vi "ATECC2 System Designer.vi"() -> ()   [LabVIEW 2023]
uses:
  <vilib>/ErrorRing/Error Ring.xnode
  Option Type Defs/Rack.ctl
  Option Type Defs/Full System Configuration.ctl
  Option Type Defs/Middle Rail.ctl
  Option Type Defs/Ballast.ctl
  Option Type Defs/Rear Panel IO Configuration.ctl
  Option Type Defs/Rear Panel IO.ctl
  Option Type Defs/Front Panel IO.ctl
  Option Type Defs/Front Door.ctl
  Option Type Defs/Miscellaneous Options.ctl
  <vilib>/Utility/sysdir.llb/System Directory Type.ctl
  Option Type Defs/Filler Panel Color.ctl
  Option Type Defs/Screw Types.ctl
  Option Type Defs/Accessories.ctl
  Option Type Defs/Parts List.ctl
panel:
  out "CSV-friendly String":string
  out "Parts List":T1[](array[typedef])
  out "Current Configuration":T2={"Rack"=enum."15U; 1-Phase; 16A; 100-240V", "Middle Rail"=enum."None", "Ballast"={"Main"=0, "Small"=0, "Side"=0}, "Front Panel I/O"={"EMO Button"=FALSE, "USB 3.0"=FALSE, "Display"=FALSE, "1st USB 2.0"=FALSE, "2nd USB 2.0"=FALSE, "Ethernet 3"=FALSE, "EMO Extension (3rd Party)"=FALSE, "EMO Extension (Rack In & Out)"=FALSE, "Aux Dual C13 QAC Outlets"=FALSE, "Residual-current Circuit Breaker"=FALSE, "Serial"=FALSE, "GPIB"=FALSE}, "Rear Panel I/O"={"Rear Panel I/O Configuration"=enum."Blank Panel", "EMO Button"=FALSE, "Power, Status & Banana Ground"=FALSE, "Ethernet 2"=FALSE, "Display"=FALSE, "USB 3.0"=FALSE, "DIO"=FALSE, "GPIB"=FALSE, "Aux Dual C13 QAC Outlets"=FALSE, "Residual-current Circuit Breaker"=FALSE, "Serial"=FALSE, "SMA"=FALSE}, "Miscellaneous Options"={"Eyebolts"=FALSE, "Tower Light"=FALSE, "Top/Side Monitor Mount Kit"=FALSE, "24\" Monitor"=FALSE, "Keyboard & Mouse"=FALSE, "Secondary Ethernet Switch"=FALSE, "Extra USB Hub"=FALSE, "USB-6509"=FALSE, "Front Door"=enum."38U (Solid) IG", "Primary Ethernet Switch"=enum."Item 0", "Use Posture"=enum."Item 0"}, "Accessories"={"Screw Type"=enum."10-32", "Cage Nuts & Screws"=0.0, "Filler Panel Color"=enum."Interface Gray", "1U"=0.0, "2U"=0.0, "3U"=0.0}} {"Ballast"."Side" max=5 step=1; "Ballast"."Small" max=5 step=1; "Ballast"."Main" max=5 step=1}
  in  "Full System Configuration":T2={"Rack"=enum."15U; 1-Phase; 16A; 100-240V", "Middle Rail"=enum."None", "Ballast"={"Main"=0, "Small"=0, "Side"=0}, "Front Panel I/O"={"EMO Button"=FALSE, "USB 3.0"=FALSE, "Display"=FALSE, "1st USB 2.0"=FALSE, "2nd USB 2.0"=FALSE, "Ethernet 3"=FALSE, "EMO Extension (3rd Party)"=FALSE, "EMO Extension (Rack In & Out)"=FALSE, "Aux Dual C13 QAC Outlets"=FALSE, "Residual-current Circuit Breaker"=FALSE, "Serial"=FALSE, "GPIB"=FALSE}, "Rear Panel I/O"={"Rear Panel I/O Configuration"=enum."Blank Panel", "EMO Button"=FALSE, "Power, Status & Banana Ground"=FALSE, "Ethernet 2"=FALSE, "Display"=FALSE, "USB 3.0"=FALSE, "DIO"=FALSE, "GPIB"=FALSE, "Aux Dual C13 QAC Outlets"=FALSE, "Residual-current Circuit Breaker"=FALSE, "Serial"=FALSE, "SMA"=FALSE}, "Miscellaneous Options"={"Eyebolts"=FALSE, "Tower Light"=FALSE, "Top/Side Monitor Mount Kit"=FALSE, "24\" Monitor"=FALSE, "Keyboard & Mouse"=FALSE, "Secondary Ethernet Switch"=FALSE, "Extra USB Hub"=FALSE, "USB-6509"=FALSE, "Front Door"=enum."38U (Solid) IG", "Primary Ethernet Switch"=enum."Item 0", "Use Posture"=enum."Item 0"}, "Accessories"={"Screw Type"=enum."10-32", "Cage Nuts & Screws"=0.0, "Filler Panel Color"=enum."Interface Gray", "1U"=0.0, "2U"=0.0, "3U"=0.0}} {"Ballast"."Side" max=5 step=1; "Ballast"."Small" max=5 step=1; "Ballast"."Main" max=5 step=1}
  # "1 DC 600 per AC PDU in system\n1 DC1200 per AC PDU in system"
  # "Rear panel I/O: Select one of the three major part numbers (fully, partial, blank).\nIf yoiu want custom, select the far right main panel and chose your piece-meal parts from the table below the Rear I/O secion."
  # "Front panel I/O just needs individual part numbers for I/O sub panels."
  # "The 15U version \"fully poipulate panel\" uses the DIO version, not the C13 version. If they wanbt the C13 version, they need to build it from a custom panel."
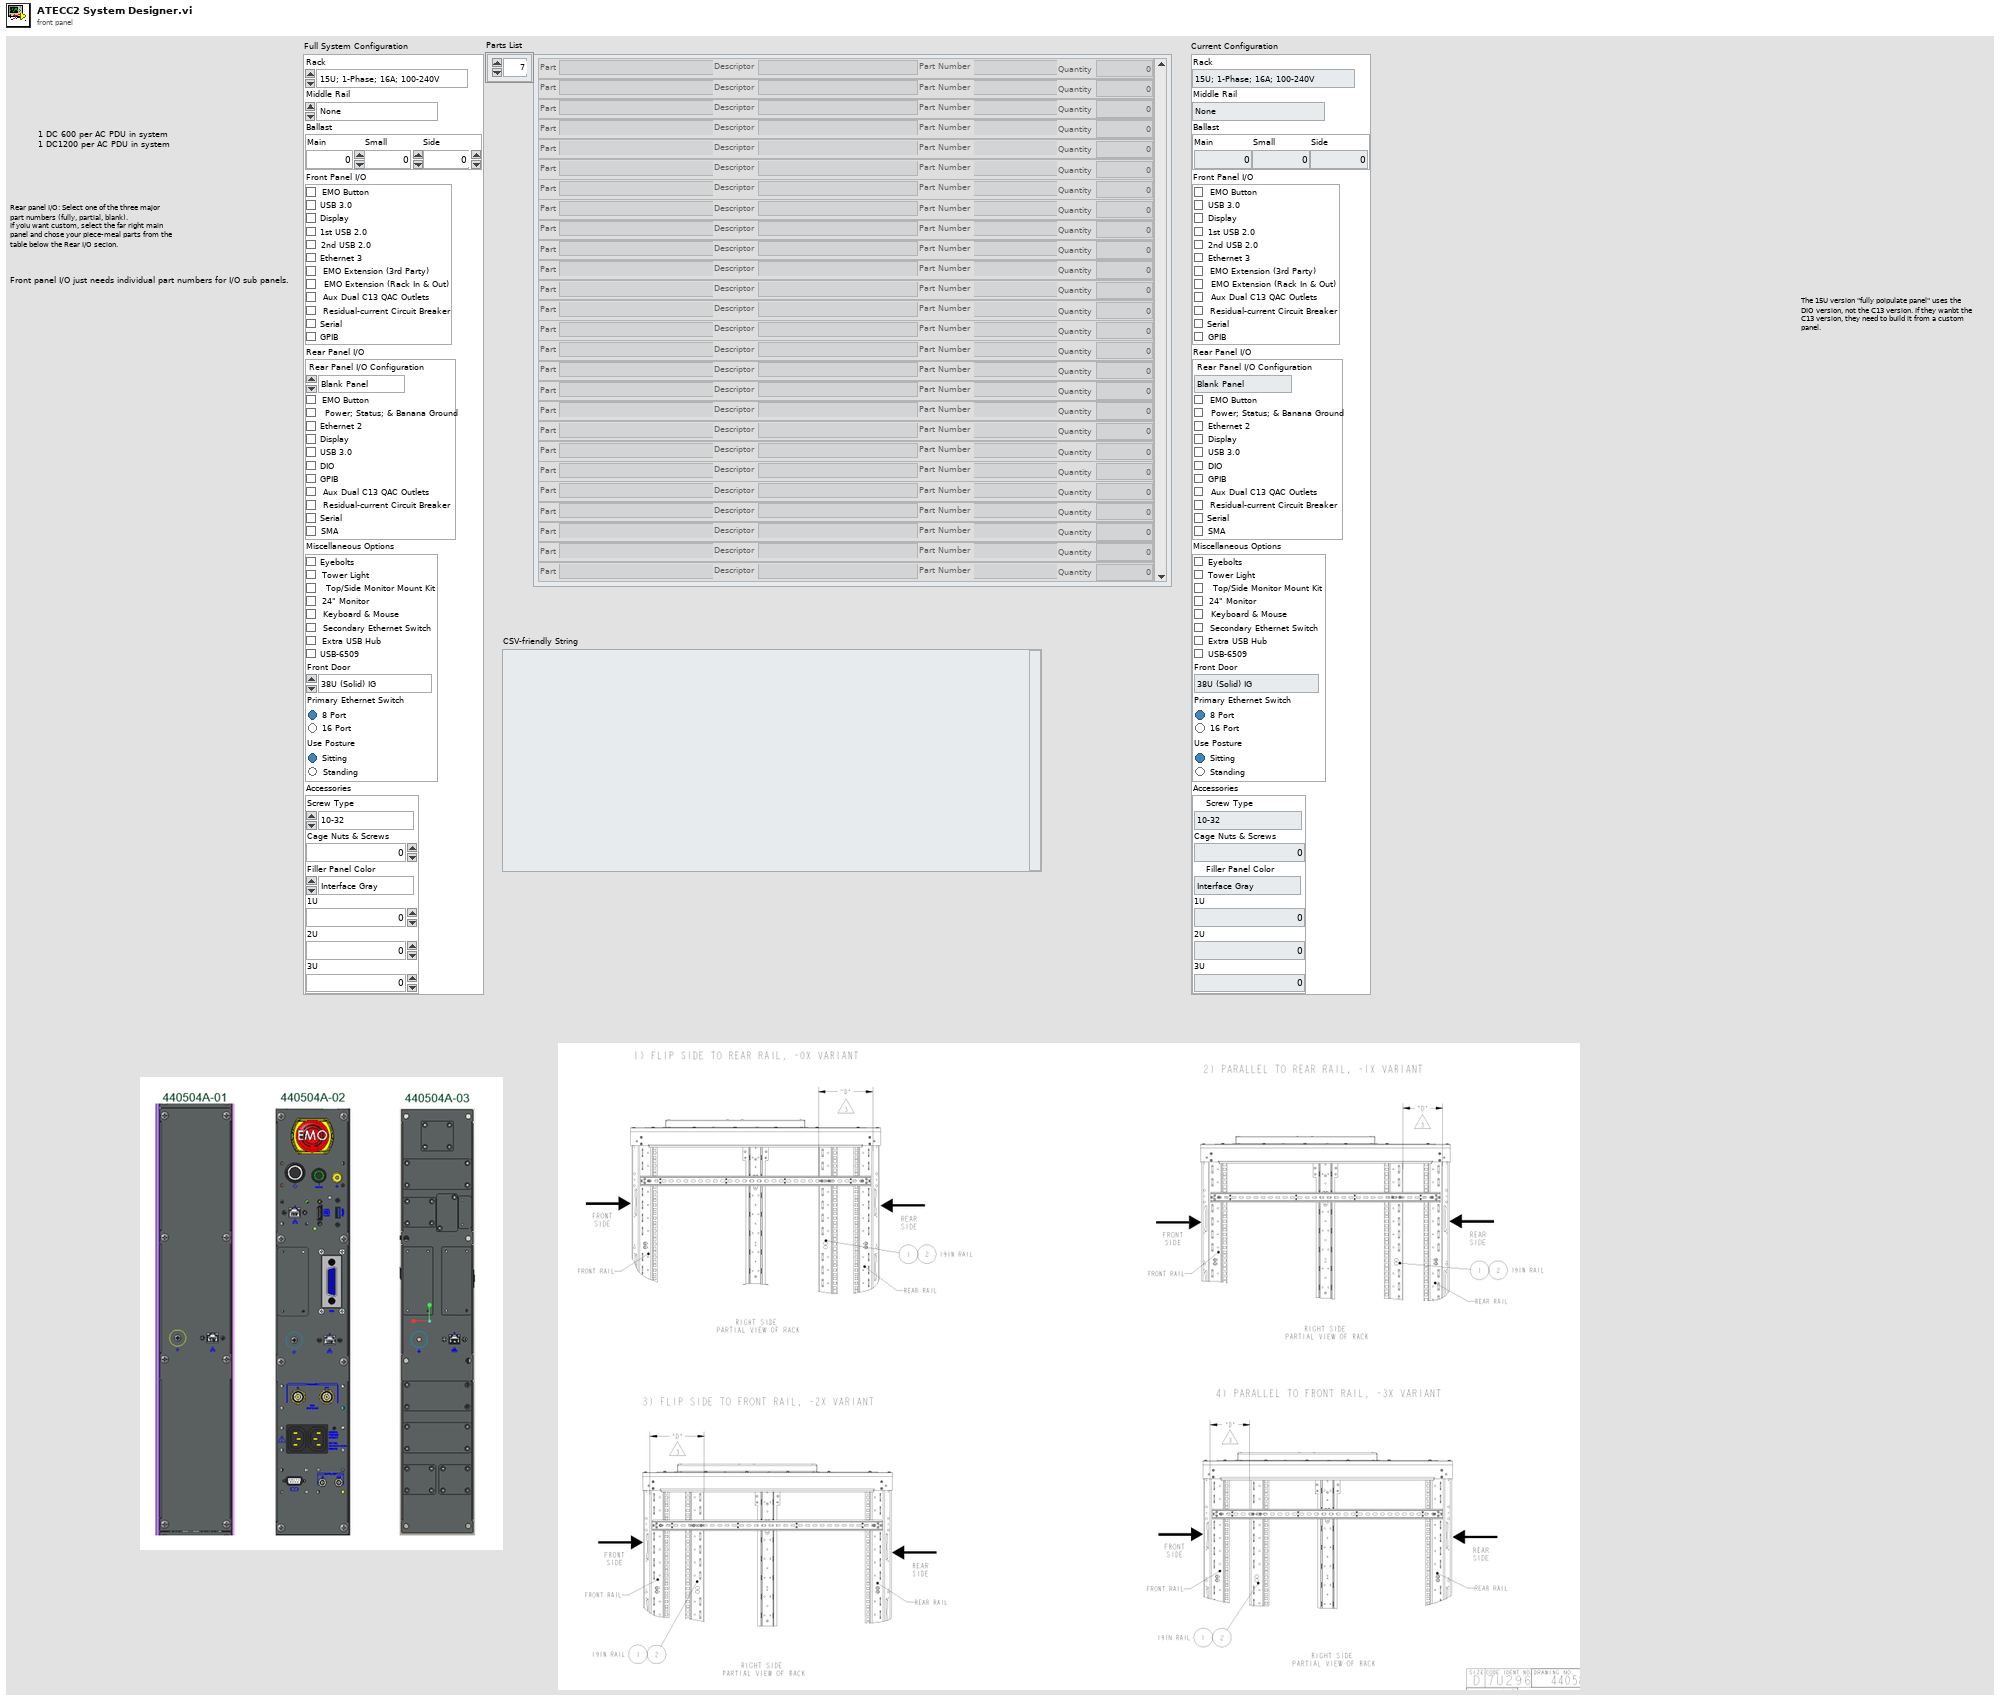
[diagram p1: front panel]
types:
  T1 = typedef "Parts List.ctl" = cluster{"Part":string, "Descriptor":string, "Part Number":string, "Quantity":dbl}
  T2 = typedef "Full System Configuration.ctl" = cluster{"Rack":T3, "Middle Rail":T4, "Ballast":T5, "Front Panel I/O":T6, "Rear Panel I/O":T7, "Miscellaneous Options":T9, "Accessories":T11}
  T3 = typedef "Rack.ctl" = enum16{"15U; 1-Phase; 16A; 100-240V", "15U; 1-Phase; 24A; 100-240V", "38U; 3-Phase Delta; 50A; 200-240V", "38U; 1-Phase; 24A; 100-120V", "38U; 3-Phase Wye; 50A; 200-240V", "38U; 3-Phase Delta; 50A; 380-480V", "38U; 3-Phase Delta; 32A; 200-240V", "38U; 3-Phase Wye; 16A; 100-240V", "44U; 1-Phase; 24A; 100-240V", "44U; 3-Phase Delta; 32A; 200-240V"}
  T4 = typedef "Middle Rail.ctl" = enum16{"None", "Flip Side Rear; D=168.83mm", "Parallel Rear; D=145mm", "Flip Side Front; D=145mm", "Parallel Front; D=145mm"}
  T5 = typedef "Ballast.ctl" = cluster{"Main":u16, "Small":u16, "Side":u16}
  T6 = typedef "Front Panel IO.ctl" = cluster{"EMO Button":bool, "USB 3.0":bool, "Display":bool, "1st USB 2.0":bool, "2nd USB 2.0":bool, "Ethernet 3":bool, "EMO Extension (3rd Party)":bool, "EMO Extension (Rack In & Out)":bool, "Aux Dual C13 QAC Outlets":bool, "Residual-current Circuit Breaker":bool, "Serial":bool, "GPIB":bool}
  T7 = typedef "Rear Panel IO.ctl" = cluster{"Rear Panel I/O Configuration":T8, "EMO Button":bool, "Power, Status & Banana Ground":bool, "Ethernet 2":bool, "Display":bool, "USB 3.0":bool, "DIO":bool, "GPIB":bool, "Aux Dual C13 QAC Outlets":bool, "Residual-current Circuit Breaker":bool, "Serial":bool, "SMA":bool}
  T8 = typedef "Rear Panel IO Configuration.ctl" = enum16{"Blank Panel", "Fully Populated Panel", "Custom Panel"}
  T9 = typedef "Miscellaneous Options.ctl" = cluster{"Eyebolts":bool, "Tower Light":bool, "Top/Side Monitor Mount Kit":bool, "24\" Monitor":bool, "Keyboard & Mouse":bool, "Secondary Ethernet Switch":bool, "Extra USB Hub":bool, "USB-6509":bool, "Front Door":T10, "Primary Ethernet Switch":enum32{"Item 0", "Item 1"}, "Use Posture":enum32{"Item 0", "Item 1"}}
  T10 = typedef "Front Door.ctl" = enum16{"None", "38U (Solid) IG", "38U (Solid) EG", "38U: Top 14U (Solid) IG", "38U (Clear) IG", "44U (Solid) IG", "44U (Solid) EG"}
  T11 = typedef "Accessories.ctl" = cluster{"Screw Type":T12, "Cage Nuts & Screws":dbl, "Filler Panel Color":T13, "1U":dbl, "2U":dbl, "3U":dbl}
  T12 = typedef "Screw Types.ctl" = enum16{"None", "M6 (Most Common)", "10-32", "12-24"}
  T13 = typedef "Filler Panel Color.ctl" = enum16{"None", "Interface Gray", "Environmental Gray"}
  T14 = typedef "System Directory Type.ctl" = i32
  T15 = enum16{"open", "replace", "create", "open or create", "replace or create", "replace or create with confirmation"}
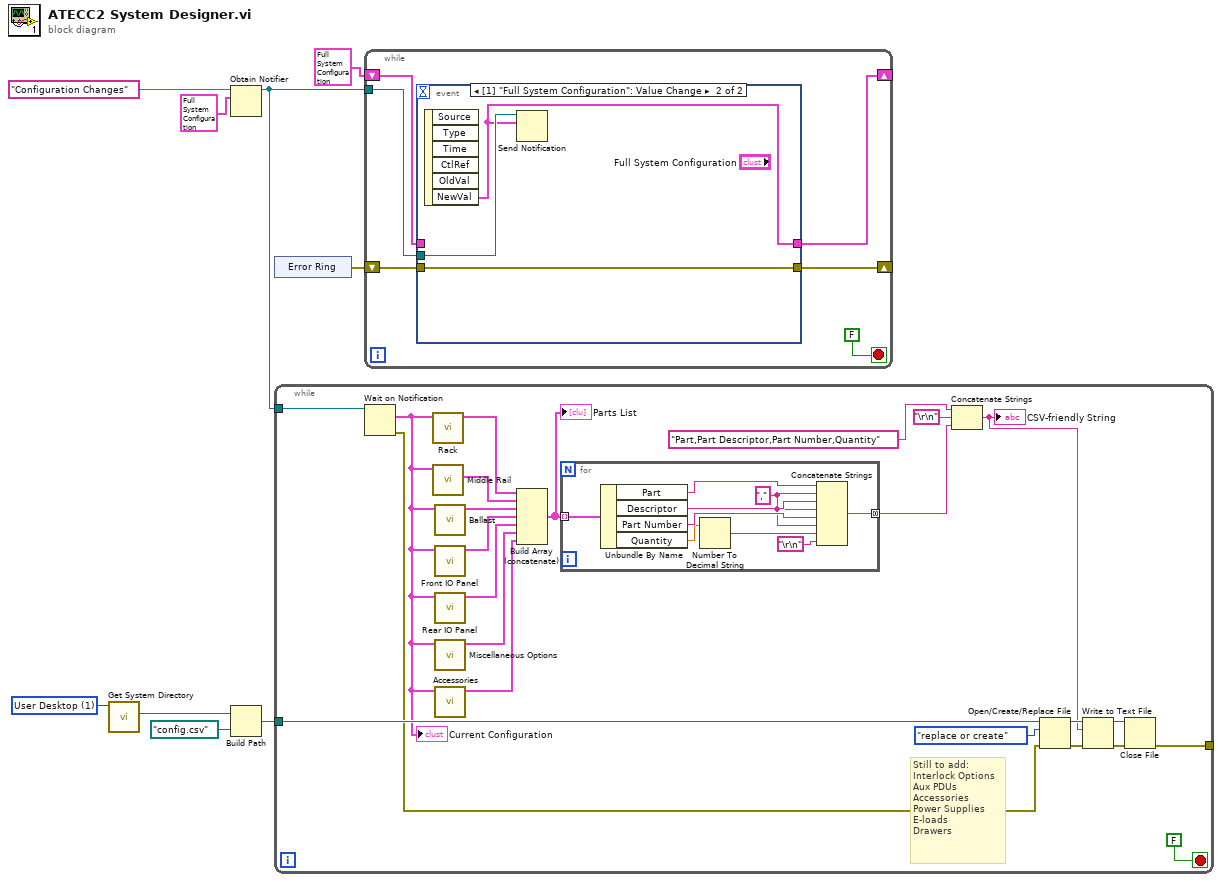
[diagram p0: block diagram]
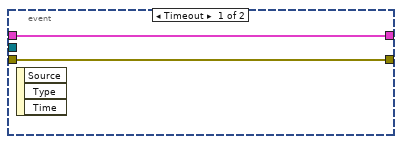
[diagram p2: hidden frame]
diagram:
  w4 = T14 1 items=["User Home"=0, "User Desktop"=1, "User Documents"=2, "User Application Data"=3, "User Preferences"=4, "User Temporary"=5, "Public Documents"=6, "Public Application Data"=7, "Public Preferences"=8, "Public Cache"=13, "System Core Libraries"=9, "System Installed Libraries"=10, "Application Files"=11, "Boot Volume Root"=12] ("system directory type")
  n1 = call <vilib>:"Get System Directory.vi"("system directory type"=w4) -> ("system directory"=w3:path)  [unwired: 10 in]
  n2 = Obtain Notifier(name (unnamed)="Configuration Changes", notification data type=T2 {"Rack"=enum."15U; 1-Phase; 16A; 100-240V", "Middle Rail"=enum."None", "Ballast"={"Main"=0, "Small"=0, "Side"=0}, "Front Panel I/O"={"EMO Button"=FALSE, "USB 3.0"=FALSE, "Display"=FALSE, "1st USB 2.0"=FALSE, "2nd USB 2.0"=FALSE, "Ethernet 3"=FALSE, "EMO Extension (3rd Party)"=FALSE, "EMO Extension (Rack In & Out)"=FALSE, "Aux Dual C13 QAC Outlets"=FALSE, "Residual-current Circuit Breaker"=FALSE, "Serial"=FALSE, "GPIB"=FALSE}, "Rear Panel I/O"={"Rear Panel I/O Configuration"=enum."Blank Panel", "EMO Button"=FALSE, "Power, Status & Banana Ground"=FALSE, "Ethernet 2"=FALSE, "Display"=FALSE, "USB 3.0"=FALSE, "DIO"=FALSE, "GPIB"=FALSE, "Aux Dual C13 QAC Outlets"=FALSE, "Residual-current Circuit Breaker"=FALSE, "Serial"=FALSE, "SMA"=FALSE}, "Miscellaneous Options"={"Eyebolts"=FALSE, "Tower Light"=FALSE, "Top/Side Monitor Mount Kit"=FALSE, "24\" Monitor"=FALSE, "Keyboard & Mouse"=FALSE, "Secondary Ethernet Switch"=FALSE, "Extra USB Hub"=FALSE, "USB-6509"=FALSE, "Front Door"=enum."38U (Solid) IG", "Primary Ethernet Switch"=enum."Item 0", "Use Posture"=enum."Item 0"}, "Accessories"={"Screw Type"=enum."10-32", "Cage Nuts & Screws"=0.0, "Filler Panel Color"=enum."Interface Gray", "1U"=0.0, "2U"=0.0, "3U"=0.0}} ("Full System Configuration")) -> (notifier out=w6:refnum<notifier>)  [unwired: 2 in, 2 out]
  n3 = Build Path(base path=w3, name or relative path=path "config.csv") -> (appended path=w1:path)
  n4 = xnode "Error Ring"() -> ("error out"=w9:errorcluster)
  n5 = while {
    tunnel: w6 -> [w32]
    tunnel: w1 -> [w19]
    tunnel: [w13] -> _
    stop <- FALSE stop-if-true
    # "Still to add:\nInterlock Options\nAux PDUs\nAccessories\nPower Supplies\nE-loads\nDrawers"
    n6 = Wait on Notification(notifier=w32) -> (notification=w10:T2, error out=w12:errorcluster)  [unwired: 3 in, 2 out]
    "Current Configuration" <- w10
    n7 = call "Rack.vi"("Full System Configuration"=w10) -> ("cluster"=w30:T1)  [unwired: 10 in]
    n8 = call "Middle Rail.vi"("Full System Configuration"=w10) -> ("cluster"=w29:T1)  [unwired: 10 in]
    n9 = call "Ballast.vi"("Full System Configuration"=w10) -> ("Array"=w28:T1[])  [unwired: 10 in]
    n10 = call "Front IO Panel.vi"("Full System Configuration"=w10) -> ("Array"=w26:T1[])  [unwired: 10 in]
    n11 = call "Rear IO Panel.vi"("Full System Configuration"=w10) -> ("Array"=w27:T1[])  [unwired: 10 in]
    n12 = call "Miscellaneous Options.vi"("Full System Configuration"=w10) -> ("Miscellaneous Options Out"=w25:T1[])  [unwired: 10 in]
    n13 = call "Accessories.vi"("Full System Configuration"=w10) -> ("Accessories Out"=w11:T1[])  [unwired: 10 in]
    n14 = Build Array (concatenate)(w30, w29, w28, w26, w27, w25, w11) -> (w24:T1[])
    "Parts List" <- w24
    n15 = for {
      tunnel: w24 -> [w41] mode=indexing
      tunnel: [w37] -> w23 mode=concatenating
      w36 = ","
      n16 = Unbundle By Name(w41) -> ("Part"=w40:string, "Descriptor"=w39:string, "Part Number"=w38:string, "Quantity"=w35:dbl)
      n17 = Number To Decimal String(number=w35) -> (decimal integer string=w34:string)  [unwired: 1 in]
      n18 = Concatenate Strings(w40, w36, w39, w36, w38, w36, w34, "\r\n") -> (w37:string)
    }
    n19 = Concatenate Strings("Part,Part Descriptor,Part Number,Quantity" ("string"), "\r\n", w23) -> (w18:string)
    "CSV-friendly String" <- w18
    n20 = Open/Create/Replace File(file path (use dialog)=w19, error in=w12, operation (0:open)=T15."replace or create") -> (refnum out=w21:refnum<file>, error out=w16:errorcluster)  [unwired: 3 in, 1 out]
    n21 = Write to Text File(file (use dialog)=w21, text=w18, error in=w16) -> (refnum out=w22:refnum<file>, error out=w17:errorcluster)  [unwired: 1 in, 1 out]
    n22 = Close File(refnum=w22, error in=w17) -> (error out=w13:errorcluster)  [unwired: 1 out]
  }
  n23 = while {
    shift-right: [w47] -> _
    shift-left: w9 -> [w46]
    shift-right: [w45] -> _
    shift-left: T2 {"Rack"=enum."15U; 1-Phase; 16A; 100-240V", "Middle Rail"=enum."None", "Ballast"={"Main"=0, "Small"=0, "Side"=0}, "Front Panel I/O"={"EMO Button"=FALSE, "USB 3.0"=FALSE, "Display"=FALSE, "1st USB 2.0"=FALSE, "2nd USB 2.0"=FALSE, "Ethernet 3"=FALSE, "EMO Extension (3rd Party)"=FALSE, "EMO Extension (Rack In & Out)"=FALSE, "Aux Dual C13 QAC Outlets"=FALSE, "Residual-current Circuit Breaker"=FALSE, "Serial"=FALSE, "GPIB"=FALSE}, "Rear Panel I/O"={"Rear Panel I/O Configuration"=enum."Blank Panel", "EMO Button"=FALSE, "Power, Status & Banana Ground"=FALSE, "Ethernet 2"=FALSE, "Display"=FALSE, "USB 3.0"=FALSE, "DIO"=FALSE, "GPIB"=FALSE, "Aux Dual C13 QAC Outlets"=FALSE, "Residual-current Circuit Breaker"=FALSE, "Serial"=FALSE, "SMA"=FALSE}, "Miscellaneous Options"={"Eyebolts"=FALSE, "Tower Light"=FALSE, "Top/Side Monitor Mount Kit"=FALSE, "24\" Monitor"=FALSE, "Keyboard & Mouse"=FALSE, "Secondary Ethernet Switch"=FALSE, "Extra USB Hub"=FALSE, "USB-6509"=FALSE, "Front Door"=enum."38U (Solid) IG", "Primary Ethernet Switch"=enum."Item 0", "Use Posture"=enum."Item 0"}, "Accessories"={"Screw Type"=enum."10-32", "Cage Nuts & Screws"=0.0, "Filler Panel Color"=enum."Interface Gray", "1U"=0.0, "2U"=0.0, "3U"=0.0}} ("Full System Configuration") -> [w44]
    tunnel: w6 -> [w42]
    stop <- FALSE stop-if-true
    n24 = event shown="[1] \"Full System Configuration\": Value Change" {
      selector: _ -> [_ _]
      dyn-events: _ -> [_ _]
      timeout: _ -> [_ _]
      tunnel: [w49 w52] -> w47
      tunnel: w46 -> [w49 w52]
      tunnel: [w48 w50] -> w45
      tunnel: w44 -> [w48 _]
      tunnel: w42 -> [_ w51]
      event Timeout {
        n25 = event-data() -> ()  [unwired: 1 in, 3 out]
      }
      event Value Change {
        n26 = event-data() -> ("NewVal"=w50:T2)  [unwired: 1 in, 5 out]
        n27 = Send Notification(notification=w50, notifier=w51) -> ()  [unwired: 1 in, 2 out]
      }
    }
  }
